vi "Get Manufacturer Device Name.vi"(8 "error in (no error)":errorcluster, 11 "FHPP in":refnum<class "FHPP.lvclass">) -> (0 "error out":errorcluster, 2 "Manufacturer Device Name":string, 3 "FHPP Out":refnum<class "FHPP.lvclass">)   [LabVIEW 2022 SP3, in "FHPP.lvclass"]
doc: "Retrieve the <b>Manufacturer Device Name</b> of the device by FCT."
uses:
  FHPP.lvclass
  FCT Request.ctl
  ReqID.ctl
  FHPP.lvclass/FHPP.ctl
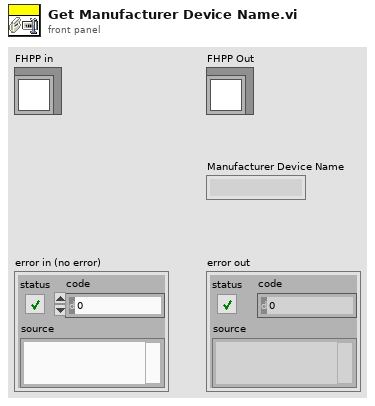
[diagram p1: front panel]
types:
  T1 = typedef "FHPP.lvclass/FCT Request.ctl" = cluster{"Request":T2, "PNU":u16, "Subindex":u16, "Data":u32}
  T2 = typedef "FHPP.lvclass/ReqID.ctl" = u8
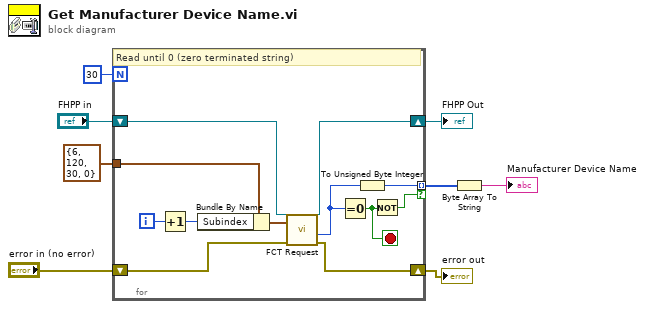
[diagram p0: block diagram]
diagram:
  n1 = for {
    N: 30 -> [_]
    tunnel: [w9] -> w7 mode=indexing if=w12
    tunnel: T1 {"Request"=6, "PNU"=120, "Subindex"=30, "Data"=0} ("Reqest") -> [w17]
    shift-right: [w10] -> w1
    shift-left: "FHPP in" -> [w20]
    shift-right: [w18] -> w4
    shift-left: "error in (no error)" -> [w19]
    i -> [w16]
    stop <- w13 stop-if-true
    # "Read until 0 (zero terminated string)"
    n2 = Increment(x=w16) -> (x+1=w15:i32)
    n3 = Bundle By Name(cluster=w17, "Subindex"=w15) -> (w14:T1)
    n4 = call-dynamic "FCT Request.vi"("error in (no error)"=w19, "Reqest"=w14, "FHPP in"=w20) -> ("error out"=w18:errorcluster, "Data"=w11:u32, "FHPP Out"=w10:refnum<class "FHPP.lvclass">)  [unwired: 5 in, 1 out]
    n5 = Equal To 0?(x=w11) -> (x = 0?=w13:bool)
    n6 = To Unsigned Byte Integer(number=w11) -> (unsigned 8bit integer=w9:u8)
    n7 = Not(x=w13) -> (.not. x?=w12:bool)
  }
  "error out" <- w4
  "FHPP Out" <- w1
  n8 = Byte Array To String(unsigned byte array=w7) -> (string=→"Manufacturer Device Name":string)
